vi "Read Path.vi"(9 "SubVI in":refnum<class "SubVI.lvclass">) -> (3 "SubVI out":refnum<class "SubVI.lvclass">, 4 "Path":path)   [LabVIEW 2014, in "SubVI.lvclass"]
uses:
  SubVI.lvclass
  SubVI.lvclass/SubVI.ctl
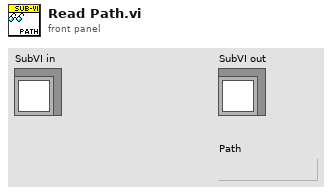
[diagram p1: front panel]
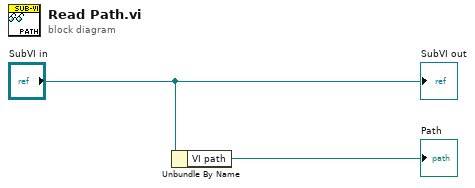
[diagram p0: block diagram]
diagram:
  n1 = Unbundle By Name("SubVI in") -> ("VI path"=→"Path":path)
  "SubVI out" <- "SubVI in"
